vi "Configure Mode.vi"(8 "error in (no error)":errorcluster, 10 "mode":T1 {"modulation mode" items=["off"=0, "internal full"=2, "internal partial"=3, "external full"=4, "external partial"=5]; "control mode" items=["Pload", "Pfwd"]}, 11 "HFP Gen in":refnum<class "PL HFP Generator.lvclass">) -> (0 "error out":errorcluster, 3 "HFP Gen out":refnum<class "PL HFP Generator.lvclass">)   [LabVIEW 2015, in "PL HFP Generator.lvclass"]
doc: "Configures power, rf output, control mode, modulation mode and SWR timer."
uses:
  PL HFP Generator.lvclass
  <vilib>/plasmapper/PL Modbus Client/PL Modbus Client.lvclass
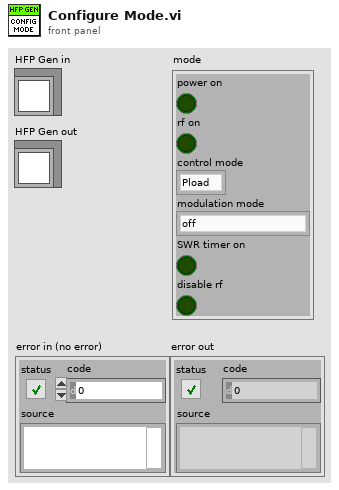
[diagram p1: front panel]
types:
  T1 = cluster{"power on":bool, "rf on":bool, "control mode":u8, "modulation mode":u8, "SWR timer on":bool, "disable rf":bool}
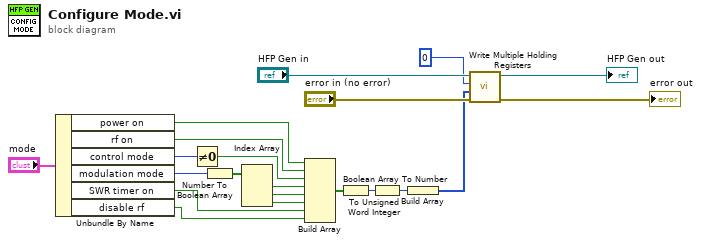
[diagram p0: block diagram]
diagram:
  n1 = Unbundle By Name("mode") -> ("power on"=w12:bool, "rf on"=w11:bool, "control mode"=w15:u8, "modulation mode"=w14:u8, "SWR timer on"=w6:bool, "disable rf"=w5:bool)
  n2 = Not Equal To 0?(x=w15) -> (x != 0?=w10:bool)
  n3 = Number To Boolean Array(number=w14) -> (Boolean array=w13:bool[])
  n4 = Index Array(array=w13) -> (element #1=w9:bool, element #2=w8:bool, element #3=w7:bool)  [unwired: 3 in]
  n5 = Build Array(w12, w11, w10, w9, w8, w7, w6, w5) -> (w4:bool[])
  n6 = Boolean Array To Number(Boolean array=w4) -> (number=w3:u32)
  n7 = To Unsigned Word Integer(number=w3) -> (unsigned 16bit integer=w2:u16)
  n8 = Build Array(w2) -> (w1:u16[])
  n9 = call <vilib>:"Write Multiple Holding Registers.vi"("error in (no error)"="error in (no error)", "values"=w1, "address"=u16 0, "MODBUS in"="HFP Gen in") -> ("error out"=→"error out":errorcluster, "MODBUS out"=→"HFP Gen out":refnum<class "PL HFP Generator.lvclass">)  [unwired: 6 in]
